vi "Init.vi"(8 "error in (no error)":errorcluster, 11 "Kasli in":refnum<class "Kasli.lvclass">) -> (0 "error out":errorcluster, 3 "Kasli out":refnum<class "Kasli.lvclass">)   [LabVIEW 2020, in "Kasli Wrapper 2.0.lvlib" / "Kasli.lvclass"]
uses:
  Kasli.lvclass
  Kasli.lvclass/Kasli.ctl
  192c0582-0505-4d32-b126-6657a1637bfb.vi
  <vilib>/Utility/config.llb/Read Key (String).vi
  <vilib>/Utility/config.llb/Read Key (Boolean).vi
  <vilib>/Comparison/Less/Less Functor/Less Functor.lvclass
  <vilib>/Utility/config.llb/NI_LVConfig.lvlib
  TALOS/TALOS_PPL.lvlibp
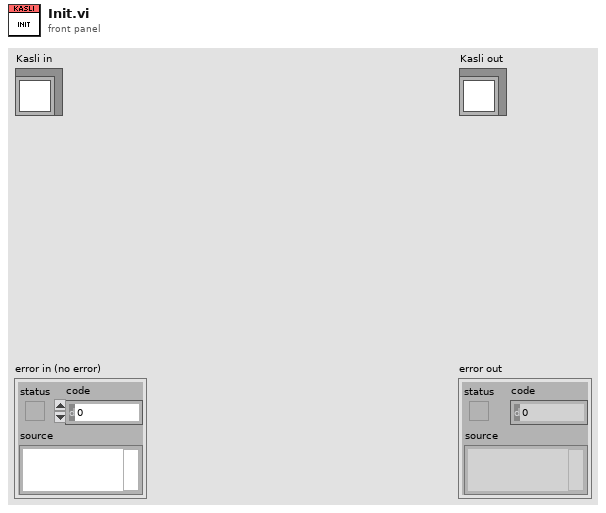
[diagram p1: front panel]
types:
  T1 = typedef "NI_LVConfig.lvlib/Config Data RefNum.ctl" = refnum<k1>
  T2 = cluster{"String":string, "value":string, "value":string}
  T3 = cluster{"String":string, "value":string, "value":string}[]
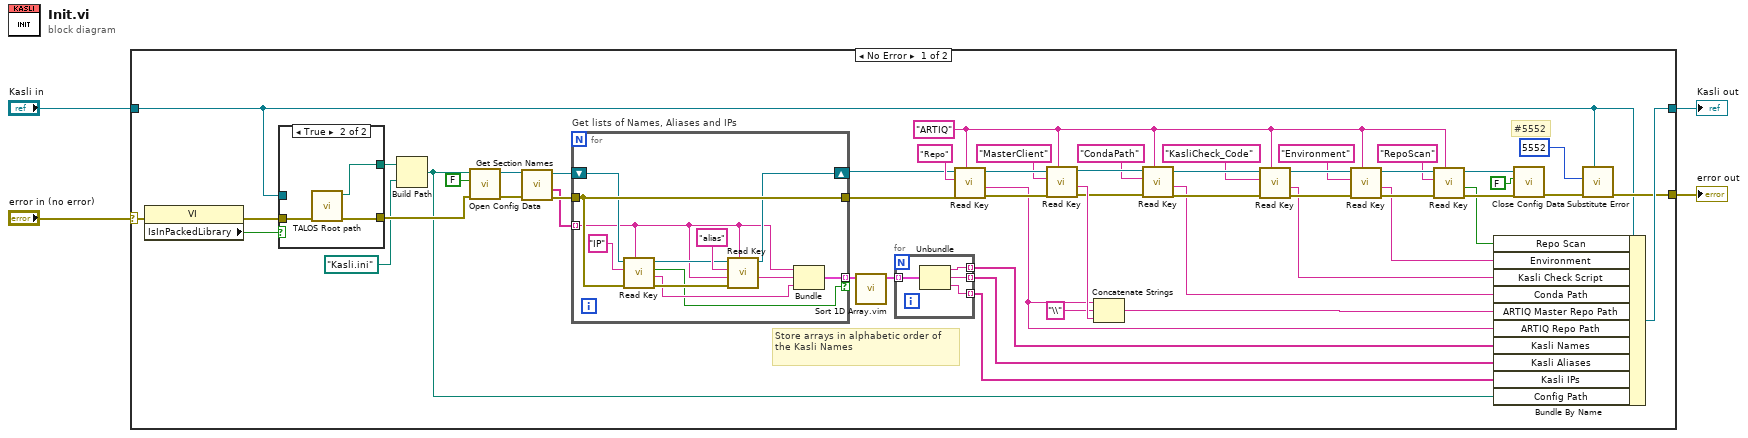
[diagram p0: block diagram]
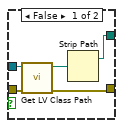
[diagram p2: hidden frame]
diagram:
  n1 = case shown="No Error" "error in (no error)" {
    selector: "error in (no error)" -> [w10 w83]
    tunnel: [w23 w83] -> w3
    tunnel: [w54 w82] -> w1
    tunnel: "Kasli in" -> [w6 w82]
    frame No Error {
      w32 = "ARTIQ" ("section")
      # "Store arrays in alphabetic order of the Kasli Names"
      # "#5552"
      n2 = property class="VI"(error in=w10) -> (error out=w8:errorcluster, "IsInPackedLibrary"=w5:bool)  [unwired: 1 in, 1 out]
      n3 = case shown="True" w5 {
        tunnel: w8 -> [w62 w65]
        tunnel: [w61 w64] -> w57
        tunnel: [w59 w63] -> w7
        tunnel: w6 -> [w58 _]
        frame False {
          n4 = call <vilib>:"Get LV Class Path.vi"("error in (no error)"=w62, "object"=w58) -> ("error out"=w61:errorcluster, "class path"=w60:path)  [unwired: 8 in]
          n5 = Strip Path(path=w60) -> (stripped path=w59:path)  [unwired: 1 out]
        }
        frame True {
          n6 = call "TALOS Root path.vi"("error in (no error)"=w65) -> ("error out"=w64:errorcluster, "TALOS Root Path"=w63:path)  [unwired: 9 in]
        }
      }
      n7 = Build Path(base path=w7, name or relative path=path "Kasli.ini") -> (appended path=w47:path)
      n8 = call <vilib>:"Open Config Data.vi"("error in (no error)"=w57, "create file if necessary (T)"=FALSE, "configuration file path"=w47) -> ("error out"=w19:errorcluster, "refnum"=w21:T1)  [unwired: 6 in, 1 out]
      n9 = call <vilib>:"Get Section Names.vi"("error in (no error)"=w19, "refnum"=w21) -> ("error out"=w17:errorcluster, "section names"=w16:string[], "refnum out"=w20:T1)  [unwired: 7 in]
      n10 = for "Get lists of Names, Aliases and IPs" {
        shift-right: [w74] -> w14
        shift-left: w20 -> [w76]
        tunnel: w16 -> [w70] mode=indexing
        tunnel: w17 -> [w77]
        tunnel: [w77] -> w15
        tunnel: [w67] -> w9 mode=indexing if=w66
        n11 = call-poly <vilib>:"Read Key.vi"("section"=w70, "error in (no error)"=w77, "key"="IP", "refnum"=w76) -> ("error out"=w73:errorcluster, "value"=w68:string, "found?"=w66:bool, "refnum out"=w71:T1)  [unwired: 4 in]
        n12 = call-poly <vilib>:"Read Key.vi"("section"=w70, "error in (no error)"=w73, "default value"=w70, "key"="alias", "refnum"=w71) -> ("value"=w69:string, "refnum out"=w74:T1)  [unwired: 3 in, 2 out]
        n13 = Bundle("String"=w70, "value"=w69, "value"=w68) -> (w67:T2)  [unwired: 1 in]
      }
      n14 = call "Sort 1D Array.vim"("unsorted array"=w9) -> ("sorted array"=w18:T3)  [unwired: 10 in]
      n15 = for {
        tunnel: w18 -> [w81] mode=indexing
        tunnel: [w80] -> w11 mode=indexing
        tunnel: [w79] -> w12 mode=indexing
        tunnel: [w78] -> w13 mode=indexing
        # "Store in sorted arrays"
        n16 = Unbundle(w81) -> ("String"=w80:string, "value"=w79:string, "value"=w78:string)
      }
      n17 = call-poly <vilib>:"Read Key.vi"("section"=w32, "error in (no error)"=w15, "key"="Repo", "refnum"=w14) -> ("error out"=w52:errorcluster, "value"=w30:string, "refnum out"=w51:T1)  [unwired: 4 in, 1 out]
      n18 = call-poly <vilib>:"Read Key.vi"("section"=w32, "error in (no error)"=w52, "key"="MasterClient", "refnum"=w51) -> ("error out"=w49:errorcluster, "value"=w56:string, "refnum out"=w50:T1)  [unwired: 4 in, 1 out]
      n19 = Concatenate Strings(w30, "\\" ("string"), w56) -> (w29:string)
      n20 = call-poly <vilib>:"Read Key.vi"("section"=w32, "error in (no error)"=w49, "key"="CondaPath", "refnum"=w50) -> ("error out"=w42:errorcluster, "value"=w28:string, "refnum out"=w43:T1)  [unwired: 4 in, 1 out]
      n21 = call-poly <vilib>:"Read Key.vi"("section"=w32, "error in (no error)"=w42, "key"="KasliCheck_Code", "refnum"=w43) -> ("error out"=w40:errorcluster, "value"=w27:string, "refnum out"=w39:T1)  [unwired: 4 in, 1 out]
      n22 = call-poly <vilib>:"Read Key.vi"("section"=w32, "error in (no error)"=w40, "key"="Environment", "refnum"=w39) -> ("error out"=w33:errorcluster, "value"=w26:string, "refnum out"=w34:T1)  [unwired: 4 in, 1 out]
      n23 = call-poly <vilib>:"Read Key.vi"("section"=w32, "error in (no error)"=w33, "key"="RepoScan", "refnum"=w34) -> ("error out"=w37:errorcluster, "value"=w25:bool, "refnum out"=w36:T1)  [unwired: 4 in, 1 out]
      n24 = Bundle By Name(cluster=w6, "Repo Scan"=w25, "Environment"=w26, "Kasli Check Script"=w27, "Conda Path"=w28, "ARTIQ Master Repo Path"=w29, "ARTIQ Repo Path"=w30, "Kasli Names"=w11, "Kasli Aliases"=w12, "Kasli IPs"=w13, "Config Path"=w47) -> (w54:refnum<class "Kasli.lvclass">)
      n25 = call <vilib>:"Close Config Data.vi"("error in (no error)"=w37, "write file if changed (T)"=FALSE, "refnum"=w36) -> ("error out"=w24:errorcluster)  [unwired: 7 in, 1 out]
      n26 = call "Substitute Error.vi"("LabVIEW Object"=w6, "error in (no error)"=w24, "Error Code"=5552) -> ("error out"=w23:errorcluster)  [unwired: 8 in]
    }
    frame Error {
    }
  }
  "error out" <- w3
  "Kasli out" <- w1
